vi "Create.vi"(8 "error in (no error)":errorcluster, 11 "Local in":refnum<class "Local.lvclass">) -> (0 "error out":errorcluster, 3 "Local out":refnum<class "Local.lvclass">)   [LabVIEW 2017, in "Local.lvclass"]
uses:
  Local.lvclass
  MatchData/MatchData.lvclass
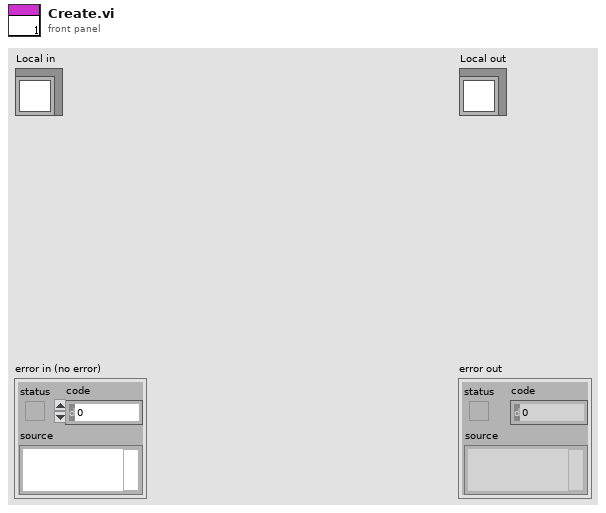
[diagram p1: front panel]
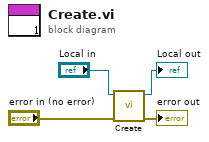
[diagram p0: block diagram]
diagram:
  n1 = call-parent "Create.vi"("error in (no error)"="error in (no error)", "MatchData in"="Local in") -> ("error out"=→"error out":errorcluster, "MatchData out"=→"Local out":refnum<class "Local.lvclass">)  [unwired: 8 in]
